vi "Video livestream 1Hz (TCP SERVER).vi"(1 "Quality":i32=750 min=0 max=1000, 2 "TCP/IP port":u16=80, 3 "VideoMode":u32, 4 "Interface name":T1="Travcam") -> (0 "Error Out":errorcluster)   [LabVIEW 2015]
doc: "This VI must be loaded when the camera server starts, and also in the list of exported VIs. This VI is not to run directly."
uses:
  <vilib>/userdefined/High Color/IMAQdx.ctl
  <vilib>/vision/driver/IMAQdx.llb/IMAQdx Camera Control Mode.ctl
  <vilib>/vision/driver/NI_Vision_Acquisition_Software.lvlib
  <resource>/objmgr/imaqdx.rc
panel:
  in  "Stop":bool
  out "Snapshot":T2(plugin-control)
  # "PN 27/08/2015"
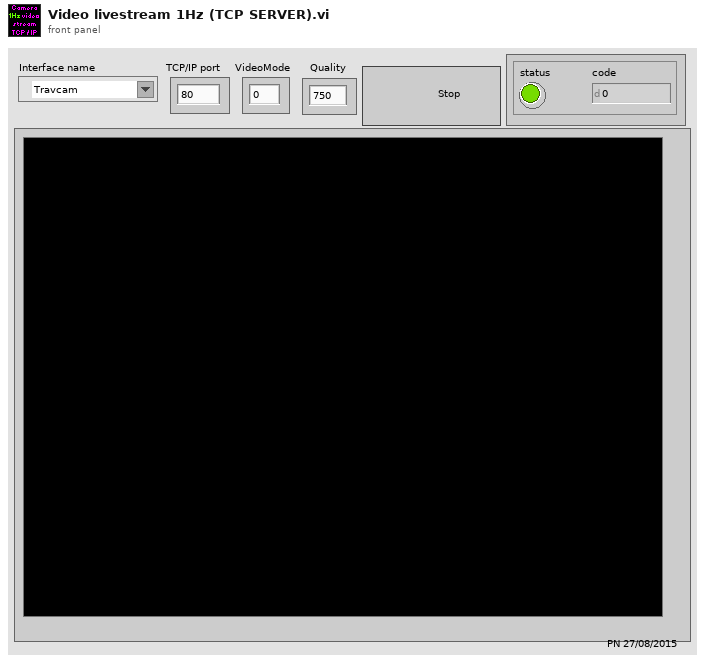
[diagram p1: front panel]
types:
  T1 = typedef "IMAQdx.ctl" = refnum<k21>
  T2 = typedef "IMAQ Image.ctl" = refnum<image>
  T3 = typedef "Image Type" = u32
  T4 = typedef "NI_Vision_Acquisition_Software.lvlib/IMAQdx Camera Control Mode.ctl" = enum32{"Controller", "Listener"}
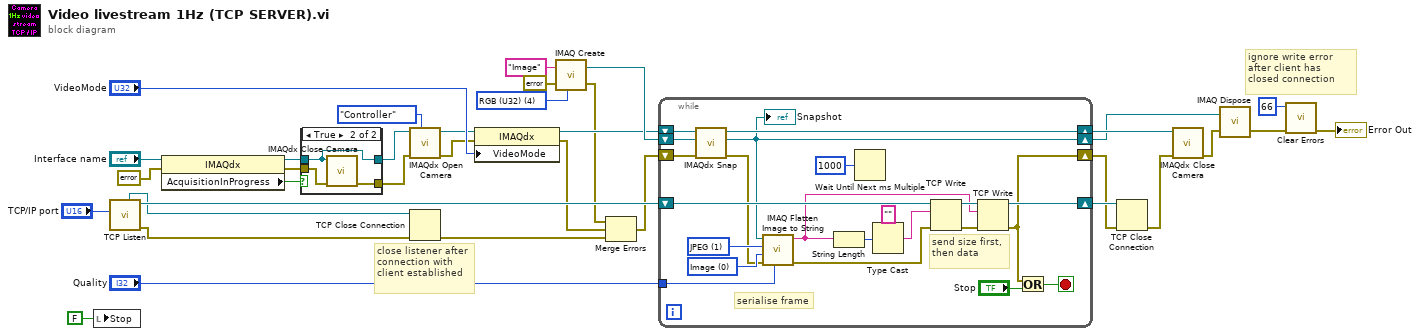
[diagram p0: block diagram]
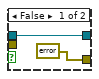
[diagram p2: hidden frame]
diagram:
  w30 = T3 4 items=["Grayscale (U8)", "Grayscale (I16)", "Grayscale (SGL)", "Complex (CSG)", "RGB (U32)", "HSL (U32)", "RGB (U64)", "Grayscale (U16)"] ("Image Type")
  # "ignore write error after client has closed connection"
  # "close listener after connection with client established"
  n1 = local write "Stop"(FALSE ("Stop")) -> ()
  n2 = call <vilib>:"TCP Listen.vi"("port"="TCP/IP port") -> ("error out"=w17:errorcluster, "connection ID"=w34:refnum<k5>, "listener ID"=w18:refnum<k5>)  [unwired: 6 in, 2 out]
  n3 = property class="IMAQdx"(reference="Interface name", error in=errorcluster {"status"=FALSE, "code"=0, "source"=""}) -> (reference out=w6:T1, error out=w4:errorcluster, "AcquisitionInProgress"=w3:bool)
  n4 = case shown="True" w3 {
    tunnel: w6 -> [w37 w38]
    tunnel: w4 -> [_ w40]
    tunnel: [errorcluster {"status"=FALSE, "code"=0, "source"=""} ("error in") w39] -> w2
    tunnel: [w37 w38] -> w5
    frame False {
    }
    frame True {
      n5 = call <vilib>:"IMAQdx Close Camera.vi"("error in"=w40, "Session In"=w38) -> ("error out"=w39:errorcluster)  [unwired: 9 in]
    }
  }
  n6 = call <vilib>:"IMAQdx Open Camera.vi"("Camera Control Mode"=IMAQdx_Camera_Control_Mode."Controller", "error in"=w2, "Session In"=w5) -> ("error out"=w24:errorcluster, "Session Out"=w23:T1)  [unwired: 7 in]
  n7 = TCP Close Connection(connection ID=w18, error in (no error)=w17) -> (error out=w16:errorcluster)  [unwired: 1 in, 1 out]
  n8 = property class="IMAQdx"(reference=w23, error in=w24, "VideoMode"="VideoMode") -> (reference out=w25:T1, error out=w21:errorcluster)
  n9 = call "IMAQ Create"("Image Name"="Image", "Image Type"=w30, "error in (no error)"=errorcluster {"status"=FALSE, "code"=0, "source"=""} ("error in")) -> ("New Image"=w29:T2, "error out"=w9:errorcluster)  [unwired: 2 in]
  n10 = Merge Errors(w9, w21, w16) -> (w20:errorcluster)
  n11 = while {
    shift-right: [w44] -> w28
    shift-left: w25 -> [w48]
    shift-right: [w43] -> w27
    shift-left: w29 -> [w47]
    shift-right: [w50] -> w14
    shift-left: w20 -> [w46]
    shift-right: [w51] -> w19
    shift-left: w34 -> [w56]
    tunnel: "Quality" -> [w41]
    stop <- w62 stop-if-true
    w59 = 1 items=["None", "JPEG", "PACKED BINARY"] ("Compression (None)")
    w60 = 0 items=["Image", "Image and Vision Info", "Reference to Image"] ("Type of Flatten (Image and Vision Info)")
    # "serialise frame"
    # "send size first, then data"
    n12 = call <vilib>:"IMAQdx Snap.vi"("error in"=w46, "Image In"=w47, "Session In"=w48) -> ("error out"=w45:errorcluster, "Image Out"=w43:T2, "Session Out"=w44:T1)  [unwired: 6 in]
    "Snapshot" <- w43
    n13 = call "IMAQ Flatten Image to String"("Quality (750)"=w41, "error in (no error)"=w45, "Type of Flatten (Image and Vision Info)"=w60, "Compression (None)"=w59, "Image"=w43) -> ("error out"=w54:errorcluster, "Data String"=w49:string)  [unwired: 5 in]
    n14 = String Length(string=w49) -> (length=w58:i32)
    n15 = Wait Until Next ms Multiple(millisecond multiple=u32 1000) -> ()  [unwired: 1 out]
    n16 = Type Cast(type="", x=w58) -> (*(type *) &x=w55:string)
    n17 = TCP Write(connection ID=w56, data in=w55, error in (no error)=w54) -> (connection ID out=w52:refnum<k5>, error out=w53:errorcluster)  [unwired: 1 in, 1 out]
    n18 = TCP Write(connection ID=w52, data in=w49, error in (no error)=w53) -> (connection ID out=w51:refnum<k5>, error out=w50:errorcluster)  [unwired: 1 in, 1 out]
    n19 = Or(x=w50, y="Stop") -> (x .or. y?=w62:bool)
  }
  n20 = TCP Close Connection(connection ID=w19, error in (no error)=w14) -> (error out=w13:errorcluster)  [unwired: 1 in, 1 out]
  n21 = call <vilib>:"IMAQdx Close Camera.vi"("error in"=w13, "Session In"=w28) -> ("error out"=w26:errorcluster)  [unwired: 9 in]
  n22 = call "IMAQ Dispose"("Image"=w27, "error in (no error)"=w26) -> ("error out"=w10:errorcluster)  [unwired: 4 in]
  n23 = call <vilib>:"Clear Errors.vi"("error in (no error)"=w10, "specific error code to clear (0: all)"=66) -> ("error out"=→"Error Out":errorcluster)  [unwired: 4 in, 1 out]
